vi "Do.vi"(8 "error in (no error)":errorcluster, 10 "Actor in":refnum<class "Actor.lvclass">, 11 "1_StartStopServer Msg in":refnum<class "1_StartStopServer Msg.lvclass">) -> (0 "error out":errorcluster, 2 "Actor out":refnum<class "Actor.lvclass">)   [LabVIEW 2018, in "MQTT_Server_Actor.lvlib" / "1_StartStopServer Msg.lvclass"]
doc: "(<B>Filename</B>: Actor Framework.lvlib:Message.lvclass:Do.vi)\n\nDefines what a message does when it is received by an actor. Generally, a message instructs an actor to invoke one of its methods. By default, this method does nothing. A child class must override it to define behavior. Create a child class by using the Actor Framework Message Maker dialog box."
uses:
  1_StartStopServer Msg.lvclass
  <vilib>/ActorFramework/Actor/Actor.lvclass
  MQTT_Server_Actor/MQTT_Server_Actor.lvclass
  D:/Program Files (x86)/National Instruments/LabVIEW 2018/vi.lib/ActorFramework/Actor/Actor.lvclass
  1_StartStopServer Msg.lvclass/1_StartStopServer Msg.ctl
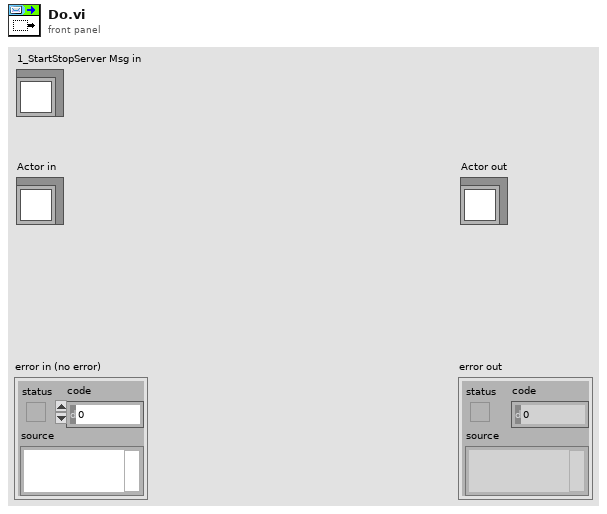
[diagram p1: front panel]
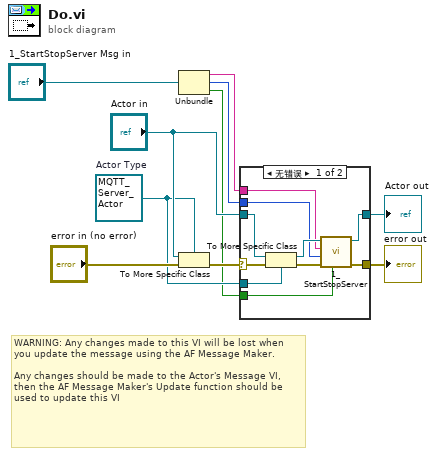
[diagram p0: block diagram]
diagram:
  w5 = refnum<class "MQTT_Server_Actor.lvclass"> refnum  # Actor Type
  # "WARNING: Any changes made to this VI will be lost when you update the message using the AF Message Maker.\n\nAny changes should be made to the Actor's Message VI, then the AF Message Maker's Update function should be used to update this VI"
  n1 = Unbundle("1_StartStopServer Msg in") -> (w4:string, w3:u16, w2:bool)
  n2 = To More Specific Class ("转换为特定的类")(target class=w5, reference="Actor in", error in="error in (no error)") -> (error out=w9:errorcluster)  [unwired: 1 out]
  n3 = case shown="无错误" w9 {
    selector: w9 -> [w20 w22]
    tunnel: [w11 w22] -> w8
    tunnel: [w12 w21] -> w7
    tunnel: "Actor in" -> [w19 w21]
    tunnel: w5 -> [w18 _]
    tunnel: w4 -> [w15 _]
    tunnel: w3 -> [w14 _]
    tunnel: w2 -> [w13 _]
    frame No Error {
      n4 = To More Specific Class ("Actor Cast")(target class=w18, reference=w19, error in=w20) -> (specific class reference=w17:refnum<class "MQTT_Server_Actor.lvclass">, error out=w16:errorcluster)
      n5 = call "1_StartStopServer.vi"("T:start"=w13, "error in (no error)"=w16, "remote port (80)"=w14, "address (localhost)"=w15, "MQTT_Server_Actor 输入"=w17) -> ("error out"=w11:errorcluster, "MQTT_Server_Actor 输出"=w12:refnum<class "MQTT_Server_Actor.lvclass">)  [unwired: 5 in]
    }
    frame Error {
    }
  }
  "error out" <- w8
  "Actor out" <- w7
